vi "Ejercicio 3.3.vi"() -> ()   [LabVIEW 2020]
panel:
  out "XY Graph":cluster{dbl[], dbl[]}(graph)
  in  "B":dbl
  in  "A":dbl
  out "Array":dbl[](array[numeric])
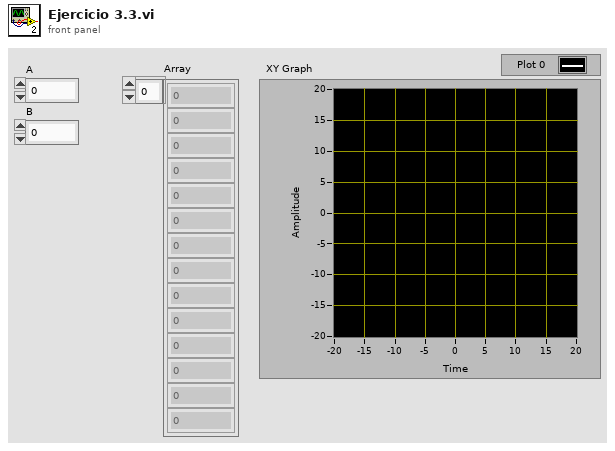
[diagram p1: front panel]
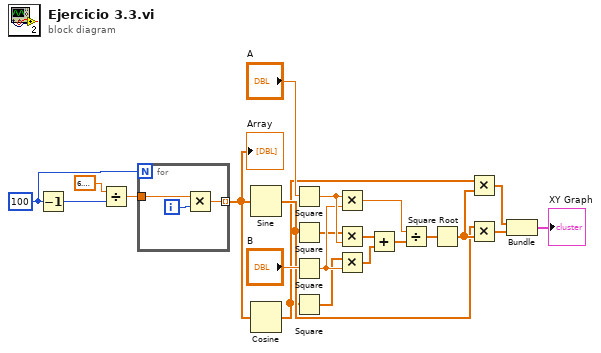
[diagram p0: block diagram]
diagram:
  w20 = 100 ("x")
  n1 = Decrement(x=w20) -> (x-1=w22:i32)
  n2 = Divide(x=6.283185307179586, y=w22) -> (x/y=w19:dbl)
  n3 = for {
    N: w20 -> [_]
    tunnel: w19 -> [w25]
    tunnel: [w23] -> w18 mode=indexing
    i -> [w24]
    n4 = Multiply(x=w25, y=w24) -> (x*y=w23:dbl)
  }
  "Array" <- w18
  n5 = Sine(x=w18) -> (sin(x)=w5:dbl[])
  n6 = Cosine(x=w18) -> (cos(x)=w4:dbl[])
  n7 = Square(x="A") -> (x^2=w15:dbl)
  n8 = Square(x=w5) -> (x^2=w12:dbl[])
  n9 = Square(x="B") -> (x^2=w14:dbl)
  n10 = Square(x=w4) -> (x^2=w13:dbl[])
  n11 = Multiply(x=w15, y=w14) -> (x*y=w8:dbl)
  n12 = Multiply(x=w12, y=w15) -> (x*y=w11:dbl[])
  n13 = Multiply(x=w13, y=w14) -> (x*y=w10:dbl[])
  n14 = Add(x=w11, y=w10) -> (x+y=w9:dbl[])
  n15 = Divide(x=w8, y=w9) -> (x/y=w7:dbl[])
  n16 = Square Root(x=w7) -> (sqrt(x)=w6:dbl[])
  n17 = Multiply(x=w4, y=w6) -> (x*y=w2:dbl[])
  n18 = Multiply(x=w5, y=w6) -> (x*y=w3:dbl[])
  n19 = Bundle(w2, w3) -> (→"XY Graph":cluster{dbl[], dbl[]})  [unwired: 1 in]
